vi "Draw Waveforms.vi"(8 "Error In (no Error) In":errorcluster, 10 "Display State In":T1={"Show Axes"=FALSE, "Show Y=0"=FALSE, "Controls"={"Type"=enum."Sine", "Periods"=0.0, "Points"=0, "Offset"=0.0, "Amplitdue"=0.0, "Phase"=0.0, "func"=""}, "Show Current Location"=FALSE, "Current Location"=0, "dt"=0.0, "t0"=timestamp(0 s since 1904-01-01), "Format and Units"="%_3p"} caption="State", 11 "Data In":T4) -> (0 "Error Out":errorcluster, 2 "Display State Out":T1={"Show Axes"=FALSE, "Show Y=0"=FALSE, "Controls"={"Type"=enum."Sine", "Periods"=0.0, "Points"=0, "Offset"=0.0, "Amplitdue"=0.0, "Phase"=0.0, "func"=""}, "Show Current Location"=FALSE, "Current Location"=0, "dt"=0.0, "t0"=timestamp(0 s since 1904-01-01), "Format and Units"="%_3p"} caption="State", 3 "Array Out":T4[](array[typedef]))   [LabVIEW 2018, in "Waveform Control.xctl"]
doc: "Creates an array of waveforms based on the input waveform + waveforms for the y=0 line and the current position marker if these are turned on in the XControl state cluster"
uses:
  Waveform Control.xctl
  Controls/Data.ctl
  Controls/Waveform State.ctl
  FP Controls.ctl
  Function Types.ctl
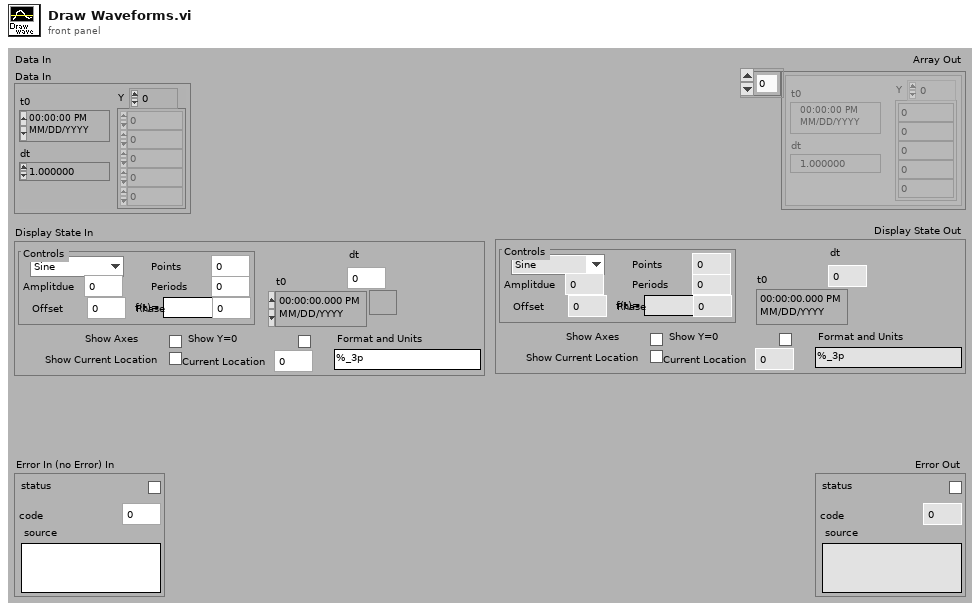
[diagram p1: front panel]
types:
  T1 = typedef "Waveform Control.xctl/Waveform State.ctl" = cluster{"Show Axes":bool, "Show Y=0":bool, "Controls":T2, "Show Current Location":bool, "Current Location":i32, "dt":dbl, "t0":timestamp, "Format and Units":string}
  T2 = typedef "Waveform Control.xctl/FP Controls.ctl" = cluster{"Type":T3, "Periods":dbl, "Points":i32, "Offset":dbl, "Amplitdue":dbl, "Phase":dbl, "func":string}
  T3 = typedef "Waveform Control.xctl/Function Types.ctl" = enum16{"Level", "Sine", "Triangle", "Ramp", "Saw Tooth", "Square", "Function"}
  T4 = typedef "Waveform Control.xctl/Data.ctl" = waveform(dbl)
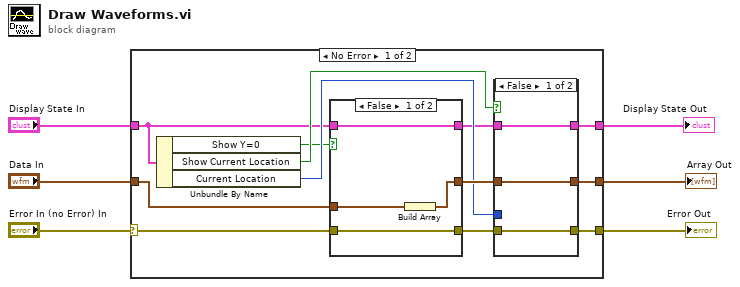
[diagram p0: block diagram]
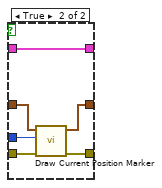
[diagram p2: hidden frame]
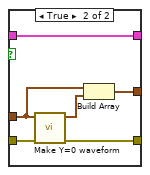
[diagram p3: hidden frame]
diagram:
  n1 = case shown="No Error" "Error In (no Error) In" {
    selector: "Error In (no Error) In" -> [w12 w39]
    tunnel: [w18 _] -> w6
    tunnel: "Data In" -> [w14 _]
    tunnel: [w10 w39] -> w3
    tunnel: [w9 w38] -> w2
    tunnel: "Display State In" -> [w7 w38]
    frame No Error {
      n2 = Unbundle By Name(w7) -> ("Show Y=0"=w13:bool, "Show Current Location"=w15:bool, "Current Location"=w16:i32)
      n3 = case shown="False" w13 {
        tunnel: [w30 w37] -> w17
        tunnel: w14 -> [w31 w36]
        tunnel: w12 -> [w29 w34]
        tunnel: [w29 w33] -> w11
        tunnel: [w28 w32] -> w8
        tunnel: w7 -> [w28 w32]
        frame False {
          n4 = Build Array(w31) -> (w30:T4[])
        }
        frame True {
          n5 = call "Make Y=0 waveform.vi"("Error In (no Error) In"=w34, "Signal In"=w36) -> ("Error Out"=w33:errorcluster, "Signal Out"=w35:waveform(dbl))  [unwired: 8 out]
          n6 = Build Array(w36, w35) -> (w37:T4[])
        }
      }
      n7 = case shown="False" w15 {
        tunnel: w16 -> [_ w27]
        tunnel: w17 -> [w21 w26]
        tunnel: [w21 w25] -> w18
        tunnel: w11 -> [w20 w24]
        tunnel: [w20 w23] -> w10
        tunnel: [w19 w22] -> w9
        tunnel: w8 -> [w19 w22]
        frame False {
        }
        frame True {
          n8 = call "Draw Current Position Marker.vi"("Error In (no Error) In"=w24, "Current Location In"=w27, "Array In"=w26) -> ("Error Out"=w23:errorcluster, "Array Out"=w25:T4[])  [unwired: 7 out]
        }
      }
    }
    frame Error {
    }
  }
  "Array Out" <- w6
  "Display State Out" <- w2
  "Error Out" <- w3
